vi "SteadyServoControl.vi"(6 "New Duty Cycle":dbl, 7 "Prev Duty Cycle":dbl, 9 "Steps":i32, 10 "PWM Ref Out in":T1, 11 "Wait Time":u32) -> (2 "Numeric":dbl, 3 "PWM Ref Out out":T1)   [LabVIEW 2015]
uses:
  <vilib>/myRIO/Instrument Drivers/Onboard IO/PWM/typedefs/PWM Reference.ctl
  <vilib>/myRIO/Common/Instrument Driver Framework/Utilities/typedefs/myRIO Generic Hardware Reference.ctl
  <vilib>/myRIO/Common/Instrument Driver Framework/Utilities/typedefs/Hardware Version Enum.ctl
  <vilib>/myRIO/Common/Instrument Driver Framework/Utilities/typedefs/myRIO v1.0 Reference.ctl
  <vilib>/myRIO/Common/Instrument Driver Framework/Utilities/typedefs/Generic FPGA Reference.ctl
  <vilib>/myRIO/Common/Instrument Driver Framework/myRIO v1.0/PWM/typedefs/PWM Channels Enum.ctl
  <vilib>/myRIO/Instrument Drivers/Onboard IO/PWM/typedefs/PWM Configuration.ctl
  <vilib>/myRIO/Instrument Drivers/Onboard IO/PWM/vis/Set Duty Cycle and Frequency.vi
  <vilib>/Utility/error.llb/Error Cluster From Error Code.vi
  <vilib>/myRIO/Common/Instrument Driver Framework/myRIO v1.0/PWM/vis/myRIO v1.0 Write PWM.vi
  <vilib>/myRIO/Instrument Drivers/Onboard IO/PWM/PWM.lvlib
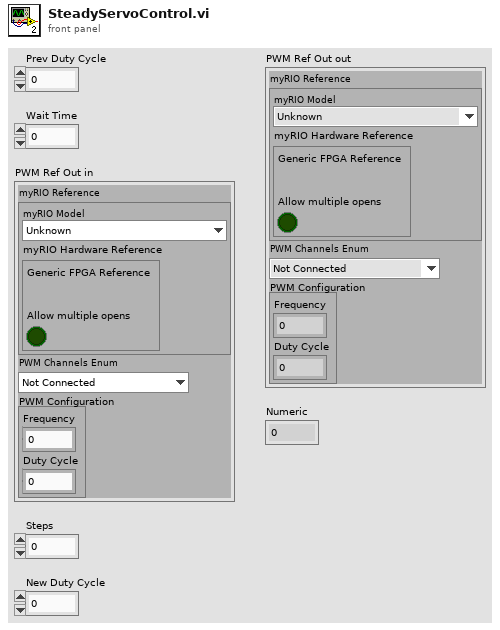
[diagram p1: front panel]
types:
  T1 = typedef "PWM.lvlib/PWM Reference.ctl" = cluster{"myRIO Reference":T2, "PWM Channels Enum":T6, "PWM Configuration":T7}
  T2 = typedef "myRIO Generic Hardware Reference.ctl" = cluster{"myRIO Model":T3, "myRIO Hardware Reference":T4}
  T3 = typedef "Hardware Version Enum.ctl" = enum16{"Unknown", "myRIO-1900", "myRIO-1950", "roboRIO"}
  T4 = typedef "myRIO v1.0 Reference.ctl" = cluster{"Generic FPGA Reference":T5, "Allow multiple opens":bool}
  T5 = typedef "Generic FPGA Reference.ctl" = refnum<k20>
  T6 = typedef "PWM Channels Enum.ctl" = enum16{"Not Connected", "C/PWM0", "C/PWM1", "A/PWM0", "A/PWM1", "A/PWM2", "B/PWM0", "B/PWM1", "B/PWM2", "PWM/PWM0", "PWM/PWM1", "PWM/PWM2", "PWM/PWM3", "PWM/PWM4", "PWM/PWM5", "PWM/PWM6", "PWM/PWM7", "PWM/PWM8", "PWM/PWM9"}
  T7 = typedef "PWM.lvlib/PWM Configuration.ctl" = cluster{"Frequency":dbl, "Duty Cycle":dbl}
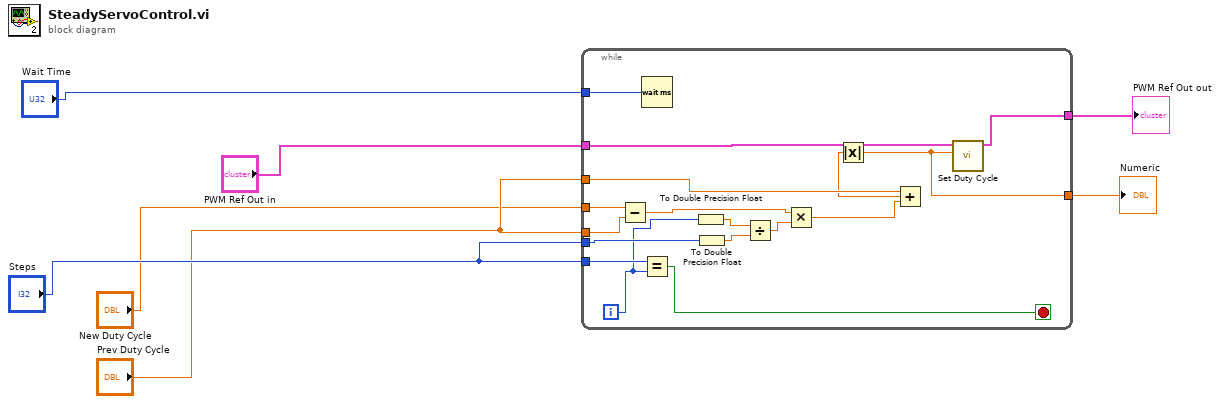
[diagram p0: block diagram]
diagram:
  n1 = while {
    tunnel: "Wait Time" -> [w24]
    tunnel: "Steps" -> [w23]
    tunnel: "PWM Ref Out in" -> [w21]
    tunnel: "New Duty Cycle" -> [w20]
    tunnel: "Prev Duty Cycle" -> [w19]
    tunnel: "Prev Duty Cycle" -> [w18]
    tunnel: "Steps" -> [w15]
    tunnel: [w9] -> w6
    tunnel: [w8] -> w7
    i -> [w14]
    stop <- w22 stop-if-true
    n2 = Subtract(x=w20, y=w19) -> (x-y=w11:dbl)
    n3 = Wait (ms)(milliseconds to wait=w24) -> ()  [unwired: 1 out]
    n4 = Equal?(x=w23, y=w14) -> (x = y?=w22:bool)
    n5 = To Double Precision Float(number=w14) -> (double precision float=w17:dbl)
    n6 = To Double Precision Float(number=w15) -> (double precision float=w16:dbl)
    n7 = Divide(x=w17, y=w16) -> (x/y=w12:dbl)
    n8 = Multiply(x=w11, y=w12) -> (x*y=w10:dbl)
    n9 = Add(x=w18, y=w10) -> (x+y=w13:dbl)
    n10 = Absolute Value(x=w13) -> (abs(x)=w9:dbl)
    n11 = call <vilib>:"Set Duty Cycle.vi"("Duty Cycle"=w9, "PWM Ref In"=w21) -> ("PWM Ref Out"=w8:T1)  [unwired: 7 in, 1 out]
  }
  "PWM Ref Out out" <- w7
  "Numeric" <- w6
